vi "ATF Storage-Data.vi"(8 "error in (no error)":errorcluster, 11 "Data FIFO Ref":T1) -> (0 "error out":errorcluster, 3 "data":string)   [LabVIEW 2022 SP3]
uses:
  RT Controls/ATF Storage-Data FIFO.ctl
panel:
  out "# elements in queue 2":i32
  out "# elements in queue":i32
  out "# elements in queue 4":i32
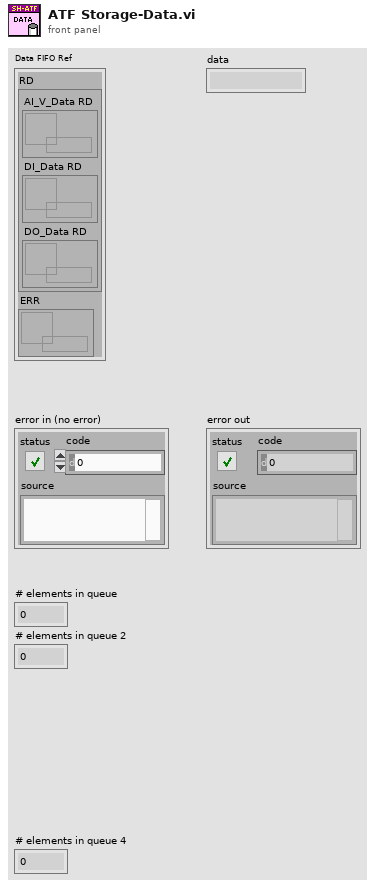
[diagram p1: front panel]
types:
  T1 = typedef "ATF Storage-Data FIFO.ctl" = cluster{"RD":cluster{"AI_V_Data RD":refnum<queue>, "DI_Data RD":refnum<queue>, "DO_Data RD":refnum<queue>}, "ERR":refnum<queue>}
  T2 = cluster{"AI_V_Data":waveform(dbl)[][], "DO_Data":waveform(dbl)[][], "DI_Data":digitalwaveform[][]}
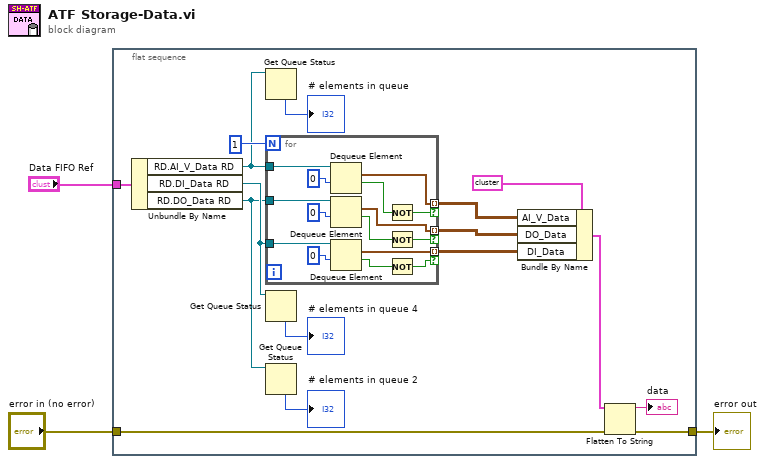
[diagram p0: block diagram]
diagram:
  n1 = flat-sequence {
    tunnel: "Data FIFO Ref" -> [w19]
    tunnel: "error in (no error)" -> [w17]
    tunnel: [w16] -> w1
    frame #0 {
      n2 = Unbundle By Name(w19) -> ("RD.AI_V_Data RD"=w10:refnum<queue>, "RD.DI_Data RD"=w13:refnum<queue>, "RD.DO_Data RD"=w7:refnum<queue>)
      n3 = Get Queue Status(queue=w10) -> (# elements in queue=→"# elements in queue":i32)  [unwired: 2 in, 7 out]
      n4 = for {
        N: 1 -> [_]
        tunnel: w13 -> [w34]
        tunnel: [w32] -> w12 mode=indexing if=w20
        tunnel: w10 -> [w30]
        tunnel: [w28] -> w11 mode=indexing if=w27
        tunnel: w7 -> [w25]
        tunnel: [w23] -> w6 mode=indexing if=w22
        n5 = Dequeue Element(queue=w30, timeout in ms (-1)=0) -> (element=w28:waveform(dbl)[], timed out?=w31:bool)  [unwired: 1 in, 2 out]
        n6 = Dequeue Element(queue=w25, timeout in ms (-1)=0) -> (element=w23:waveform(dbl)[], timed out?=w26:bool)  [unwired: 1 in, 2 out]
        n7 = Dequeue Element(queue=w34, timeout in ms (-1)=0) -> (element=w32:digitalwaveform[], timed out?=w21:bool)  [unwired: 1 in, 2 out]
        n8 = Not(x=w31) -> (.not. x?=w27:bool)
        n9 = Not(x=w26) -> (.not. x?=w22:bool)
        n10 = Not(x=w21) -> (.not. x?=w20:bool)
      }
      n11 = Get Queue Status(queue=w13) -> (# elements in queue=→"# elements in queue 4":i32)  [unwired: 2 in, 7 out]
      n12 = Get Queue Status(queue=w7) -> (# elements in queue=→"# elements in queue 2":i32)  [unwired: 2 in, 7 out]
      n13 = Bundle By Name(cluster=T2 data[100104B] ("data out"), "AI_V_Data"=w11, "DO_Data"=w6, "DI_Data"=w12) -> (w15:T2)
      n14 = Flatten To String(anything=w15, error in (no error)=w17) -> (data string=→"data":string, error out=w16:errorcluster)  [unwired: 2 in, 1 out]
    }
  }
  "error out" <- w1
